vi "Process Calculation Results.vi"(8 "error in (no error)":errorcluster, 10 "GPU Calculation Results":T1 {"Zoom Parameters"."fwidth:" format="%#_6p"; "Zoom Parameters"."f0:" format="%#_6p"}, 11 "GPU FFT Calculator in":refnum<class "GPU FFT Calculator.lvclass">) -> (0 "error out":errorcluster, 3 "GPU FFT Calculator out":refnum<class "GPU FFT Calculator.lvclass">)   [LabVIEW 2020, in "GPU FFT Calculator.lvlib" / "GPU FFT Calculator.lvclass"]
uses:
  GPU FFT Calculator.lvclass
  C:/Users/natan/Documents/G2CPU-Performance-Demo/Calculation Worker/Calculation Worker/Calculation Worker.lvclass
  C:/Program Files/National Instruments/LabVIEW 2026/vi.lib/ActorFramework/Actor/Actor.lvclass
  GPU Calculation Message.ctl
  <vilib>/Natan Biesmans/G2CPU GPU and CPU HPC Toolkit/G2CPU Libraries/Async IO/DMA Manager/DMA Manager.lvclass
  <vilib>/Natan Biesmans/G2CPU GPU and CPU HPC Toolkit/G2CPU Libraries/Arrays/1DArray/s16/1D Array s16.lvclass
  <vilib>/Natan Biesmans/G2CPU GPU and CPU HPC Toolkit/G2CPU Libraries/Arrays/1DArray/f32/1D Array f32.lvclass
  chart zoom.ctl
  GPU Metrics.ctl
  Simple UI/Simple UI/GPU Batch Results.ctl
  <vilib>/ActorFramework/Actor/Actor.lvclass/Actor.ctl
  <vilib>/ActorFramework/Message Enqueuer/Message Enqueuer.lvclass/Message Enqueuer.ctl
  Application Manager/Application Manager Messages/Update GPU UI Components Msg/Update GPU UI Components Msg.lvclass/Update GPU UI Components Msg.ctl
  Application Manager/Application Manager Messages/Update GPU Graph Msg/Update GPU Graph Msg.lvclass/Update GPU Graph Msg.ctl
  GPU FFT Calculator Messages/Stop Calculation Msg/Stop Calculation Msg.lvclass/Stop Calculation Msg.ctl
  <vilib>/ActorFramework/Message Enqueuer/Init from Existing Queue.vi
  <vilib>/ActorFramework/Message Enqueuer/Enqueue.vi
  Application Manager/Application Manager Messages/Update GPU UI Components Msg/Update GPU UI Components Msg.lvclass
  C:/Program Files/National Instruments/LabVIEW 2026/vi.lib/ActorFramework/Message/Message.lvclass
  Application Manager/Application Manager Messages/Update GPU Graph Msg/Update GPU Graph Msg.lvclass
  GPU FFT Calculator Messages/Stop Calculation Msg/Stop Calculation Msg.lvclass
  <vilib>/ActorFramework/Message Priority Queue/Priority Enqueue.vi
  <vilib>/ActorFramework/Message Enqueuer/Message Enqueuer.lvclass
  <vilib>/ActorFramework/Actor/Actor.lvclass
  Simple UI/Simple UI/Simple UI.lvclass
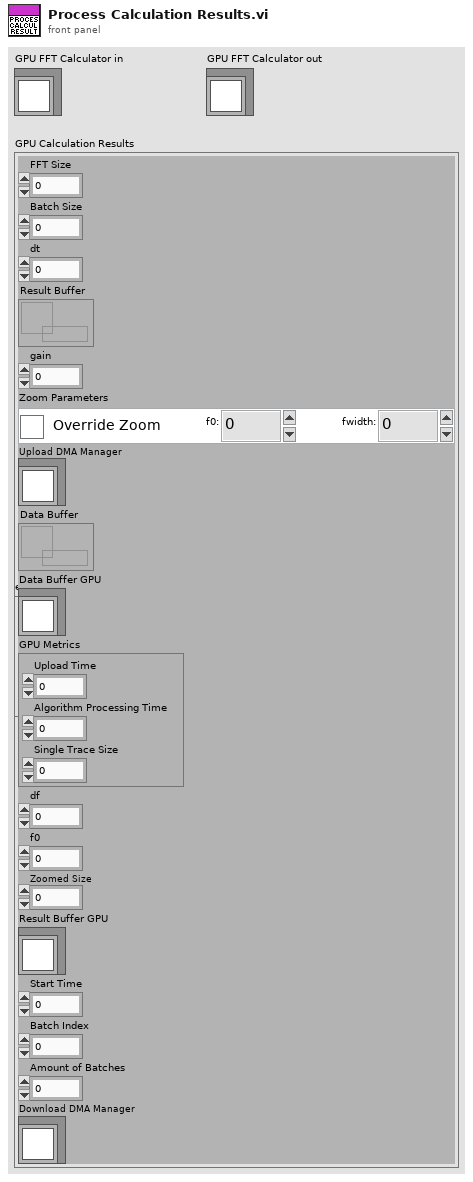
[diagram p1: front panel]
types:
  T1 = typedef "GPU FFT Calculator.lvlib/GPU FFT Calculator.lvclass/GPU Calculation Message.ctl" = cluster{"FFT Size":u64, "Batch Size":u64, "dt":dbl, "Result Buffer":refnum<data-value>, "gain":dbl, "Zoom Parameters":T2, "Upload DMA Manager":refnum<class "DMA Manager.lvclass">, "Data Buffer":refnum<data-value>, "Data Buffer GPU":refnum<class "1D Array s16.lvclass">, "GPU Metrics":T3, "df":dbl, "f0":dbl, "Zoomed Size":u64, "Result Buffer GPU":refnum<class "1D Array f32.lvclass">, "Start Time":dbl, "Batch Index":i32, "Amount of Batches":i32, "Download DMA Manager":refnum<class "DMA Manager.lvclass">}
  T2 = typedef "Simple UI.lvlib/Simple UI.lvclass/chart zoom.ctl" = cluster{"Override":bool, "f0: ":dbl, "fwidth: ":dbl}
  T3 = typedef "GPU FFT Calculator.lvlib/GPU FFT Calculator.lvclass/GPU Metrics.ctl" = cluster{"Upload Time":dbl, "Algorithm Processing Time":dbl, "Single Trace Size":u64}
  T4 = typedef "Simple UI.lvlib/Simple UI.lvclass/GPU Batch Results.ctl" = cluster{"Queue Depth":dbl, "Throughput":dbl, "Upload Speed":dbl, "Elapsed Time":dbl, "Throughput Valid":bool}
  T5 = typedef "Data Source.lvlib/Data Source.lvclass/Data Source Buffer.ctl" = refnum<data-value>
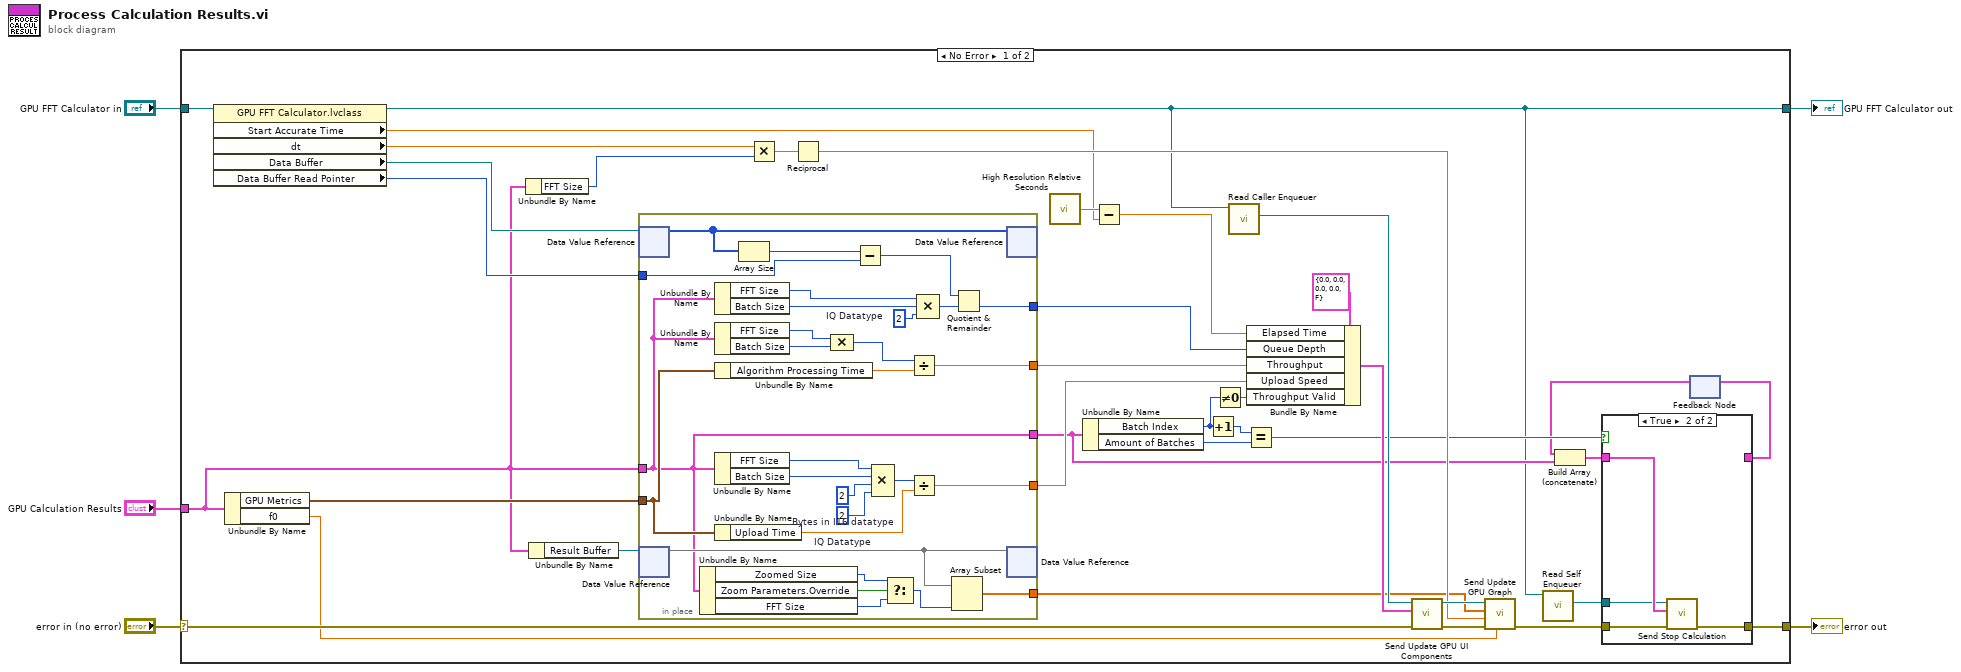
[diagram p0: block diagram]
diagram:
  n1 = case shown="No Error" "error in (no error)" {
    selector: "error in (no error)" -> [w42 w79]
    tunnel: [w10 w79] -> w4
    tunnel: [w8 w78] -> w2
    tunnel: "GPU FFT Calculator in" -> [w36 w78]
    tunnel: "GPU Calculation Results" -> [w19 _]
    frame No Error {
      n2 = property class="GPU FFT Calculator.lvclass"(reference=w36) -> (reference out=w8:refnum<class "GPU FFT Calculator.lvclass">, "Start Accurate Time"=w22:dbl, "dt"=w30:dbl, "Data Buffer"=w33:T5, "Data Buffer Read Pointer"=w34:u64)  [unwired: 1 in, 1 out]
      n3 = Unbundle By Name(w19) -> ("GPU Metrics"=w28:T3, "f0"=w20:dbl)
      n4 = Unbundle By Name(w19) -> ("FFT Size"=w24:u64)
      n5 = Unbundle By Name(w19) -> ("Result Buffer"=w27:refnum<data-value>)
      n6 = in-place {
        in-place-border: w19 -> [w47]
        in-place-border: w28 -> [w50]
        in-place-border: [w66] -> w38
        in-place-border: [w61] -> w37
        in-place-border: [w54] -> w35
        in-place-border: w34 -> [w53]
        in-place-border: [w48] -> w26
        in-place-border: [w47] -> w11
        w51 = u64 2  # IQ Datatype
        w52 = u64 2  # IQ Datatype
        w71 = u64 2  # Bytes in I16 datatype
        n7 = in-place-dvr #1(w33) -> (w60:i16[])  [unwired: 1 out]
        n8 = in-place-dvr #2(w27) -> (w49:sgl[])  [unwired: 1 out]
        n9 = Unbundle By Name(w47) -> ("Zoomed Size"=w43:u64, "Zoom Parameters.Override"=w46:bool, "FFT Size"=w45:u64)
        n10 = Unbundle By Name(w47) -> ("FFT Size"=w57:u64, "Batch Size"=w56:u64)
        n11 = Unbundle By Name(w47) -> ("FFT Size"=w64:u64, "Batch Size"=w65:u64)
        n12 = Unbundle By Name(w50) -> ("Algorithm Processing Time"=w63:dbl)
        n13 = Unbundle By Name(w47) -> ("FFT Size"=w70:u64, "Batch Size"=w69:u64)
        n14 = Unbundle By Name(w50) -> ("Upload Time"=w67:dbl)
        n15 = Array Size(array=w60) -> (size(s)=w59:i32)
        n16 = Compound Arithmetic op=MULTIPLY(w64, w65) -> (w62:u64)
        n17 = Subtract(x=w59, y=w53) -> (x-y=w58:u64)
        n18 = Compound Arithmetic op=MULTIPLY(w70, w69, w71, w52) -> (w68:u64)
        n19 = Select(t=w43, s=w46, f=w45) -> (s? t:f=w44:u64)
        n20 = Divide(x=w62, y=w63) -> (x/y=w61:dbl)
        n21 = Divide(x=w68, y=w67) -> (x/y=w66:dbl)
        n22 = Compound Arithmetic op=MULTIPLY(w57, w56, w51) -> (w55:u64)
        n23 = Array Subset(array=w49, length=w44) -> (w48:sgl[])  [unwired: 1 in]
        n24 = Quotient & Remainder(x=w58, y=w55) -> (floor(x/y)=w54:u64)  [unwired: 1 out]
        n25 = in-place-dvr #1(w60) -> ()  [unwired: 2 out]
        n26 = in-place-dvr #2(w49) -> ()  [unwired: 2 out]
      }
      n27 = Multiply(x=w30, y=w24) -> (x*y=w25:dbl)
      n28 = Reciprocal(x=w25) -> (1/x=w29:dbl)
      n29 = call <vilib>:"High Resolution Relative Seconds.vi"() -> ("relative seconds"=w23:dbl)
      n30 = Unbundle By Name(w11) -> ("Batch Index"=w6:i32, "Amount of Batches"=w17:i32)
      n31 = Subtract(x=w23, y=w22) -> (x-y=w21:dbl)
      n32 = Increment(x=w6) -> (x+1=w18:i32)
      n33 = Not Equal To 0?(x=w6) -> (x != 0?=w7:bool)
      n34 = call <vilib>:"Read Caller Enqueuer.vi"("Actor"=w8) -> ("Caller Enqueuer"=w41:refnum<class "Message Enqueuer.lvclass">)  [unwired: 10 in]
      n35 = Equal?(x=w18, y=w17) -> (x = y?=w16:bool)
      n36 = Bundle By Name(cluster=T4 {"Queue Depth"=0.0, "Throughput"=0.0, "Upload Speed"=0.0, "Elapsed Time"=0.0, "Throughput Valid"=FALSE} ("GPU UI metrics"), "Elapsed Time"=w21, "Queue Depth"=w35, "Throughput"=w37, "Upload Speed"=w38, "Throughput Valid"=w7) -> (w39:T4)
      n37 = call "Send Update GPU UI Components.vi"("error in (no error)"=w42, "GPU UI metrics"=w39, "Message Enqueuer"=w41) -> ("error out"=w31:errorcluster, "Message Enqueuer out"=w32:refnum<class "Message Enqueuer.lvclass">)  [unwired: 7 in]
      n38 = call "Send Update GPU Graph.vi"("f0"=w20, "error in (no error)"=w31, "df"=w29, "Plot"=w26, "Message Enqueuer"=w32) -> ("error out"=w15:errorcluster)  [unwired: 5 in, 1 out]
      n39 = call <vilib>:"Read Self Enqueuer.vi"("Actor"=w8) -> ("Self Enqueuer"=w9:refnum<class "Message Enqueuer.lvclass">)  [unwired: 10 in]
      n40 = feedback #3() -> (w14:T1[])  [unwired: 1 in]
      n41 = Build Array (concatenate)(w14, w11) -> (w12:T1[])
      n42 = case shown="True" w16 {
        tunnel: w15 -> [w72 w75]
        tunnel: [w73 _] -> w13
        tunnel: w12 -> [w73 w77]
        tunnel: w9 -> [_ w76]
        tunnel: [w72 w74] -> w10
        frame False {
        }
        frame True {
          n43 = call "Send Stop Calculation.vi"("error in (no error)"=w75, "appended array"=w77, "Message Enqueuer"=w76) -> ("error out"=w74:errorcluster)  [unwired: 7 in, 1 out]
        }
      }
      n44 = feedback-in #3(w13) -> ()
    }
    frame Error {
    }
  }
  "error out" <- w4
  "GPU FFT Calculator out" <- w2
